vi "TrigerDelayer_TriggerLevel&Source_Set.vi"(8 "error in (no error)":errorcluster, 10 "Trigger Level & Source":T1, 11 "VISA Refnum in":refnum<visa-resource-name>) -> (0 "error out":errorcluster, 3 "VISA Refnum out":refnum<visa-resource-name>)   [LabVIEW 2016, in "Trigger Delayer.lvlib"]
uses:
  Trigger Delayer.lvlib
  TrigerDelayer_TriggerLevel&Source_ctl.ctl
  TrigerDelayer_ctl_TriggerSource.ctl
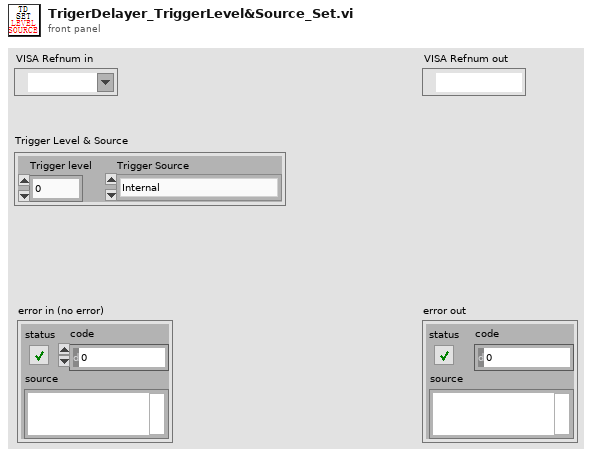
[diagram p1: front panel]
types:
  T1 = typedef "Trigger Delayer.lvlib/TrigerDelayer_TriggerLevel&Source_ctl.ctl" = cluster{"Trigger level":dbl, "Trigger Source":T2}
  T2 = typedef "Trigger Delayer.lvlib/TrigerDelayer_ctl_TriggerSource.ctl" = enum16{"Internal", "External Rising Edges", "External Falling Edges", "Single Shot External Rising Edges", "Single Shot External Falling Edges", "Single Shot", "Line"}
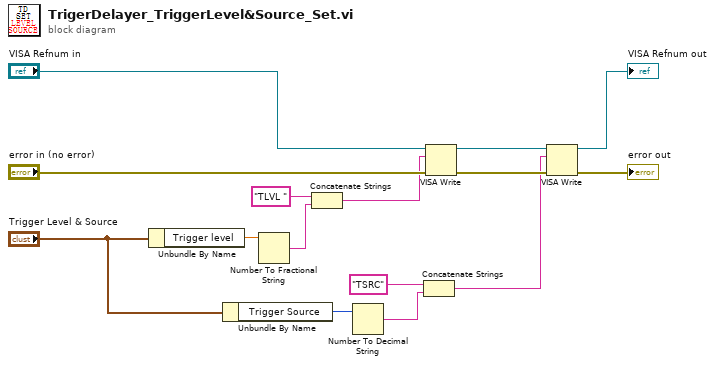
[diagram p0: block diagram]
diagram:
  n1 = Unbundle By Name("Trigger Level & Source") -> ("Trigger level"=w5:dbl)
  n2 = Unbundle By Name("Trigger Level & Source") -> ("Trigger Source"=w4:T2)
  n3 = Number To Fractional String(number=w5) -> (F-format string=w7:string)  [unwired: 3 in]
  n4 = Concatenate Strings("TLVL ", w7) -> (w8:string)
  n5 = Number To Decimal String(number=w4) -> (decimal integer string=w15:string)  [unwired: 1 in]
  n6 = Concatenate Strings("TSRC", w15) -> (w12:string)
  n7 = VISA Write(VISA resource name="VISA Refnum in", write buffer=w8, error in (no error)="error in (no error)") -> (VISA resource name out=w13:refnum<visa-resource-name>, error out=w14:errorcluster)  [unwired: 1 out]
  n8 = VISA Write(VISA resource name=w13, write buffer=w12, error in (no error)=w14) -> (VISA resource name out=→"VISA Refnum out":refnum<visa-resource-name>, error out=→"error out":errorcluster)  [unwired: 1 out]
